vi "OpenChannel.vi"(2 "error in (no error)":errorcluster, 3 "Channel ID":i32=7140 format="%_4g") -> (0 "error out":errorcluster)   [LabVIEW 2012]
doc: "Opens channel for specified ID"
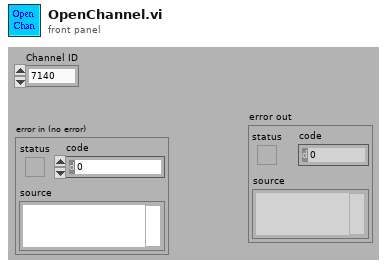
[diagram p1: front panel]
types:
  T1 = enum16{"N1911A", "Siggen", "34980a", "E4418B", "Rvp8"}
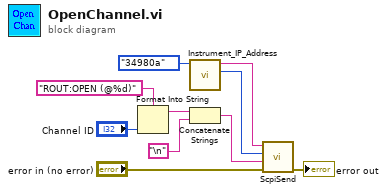
[diagram p0: block diagram]
diagram:
  n1 = Format Into String(format string="ROUT:OPEN (@%d)", "Channel ID") -> (resulting string=w8:string)  [unwired: 2 in, 1 out]
  n2 = call "Instrument_IP_Address.vi"("Instrument"=T1."34980a") -> ("Port"=w4:u16, "IP Address"=w3:string)  [unwired: 9 in]
  n3 = Concatenate Strings(w8, "\n") -> (w7:string)
  n4 = call "ScpiSend.vi"("error in (no error)"="error in (no error)", "Command"=w7, "TCP port"=w4, "IP Address"=w3) -> ("error out"=→"error out":errorcluster)  [unwired: 7 in]
